vi "Dequeue Published Result by Type.vi"(8 "error in (no error)":errorcluster, 9 "timeout in ms":i32, 10 "Result Type":T1, 11 "Mock Result Observer In":refnum<class "Mock Result Observer.lvclass">) -> (0 "error out":errorcluster, 1 "timed out?":bool, 2 "Result":T2={"Name"="", "Message"="", "Description"="", "Status"=enum."Passed", "Result Type"=enum."Method", "Execution Time"=0.0}, 3 "Mock Result Observer Out":refnum<class "Mock Result Observer.lvclass">)   [LabVIEW 2020, in "Mock Result Observer.lvclass"]
uses:
  Mock Result Observer.lvclass
  Core/Result/Result.ctl
  Core/Result/Status.ctl
  Core/Result/Type.ctl
  Core/Result/Result.lvlib
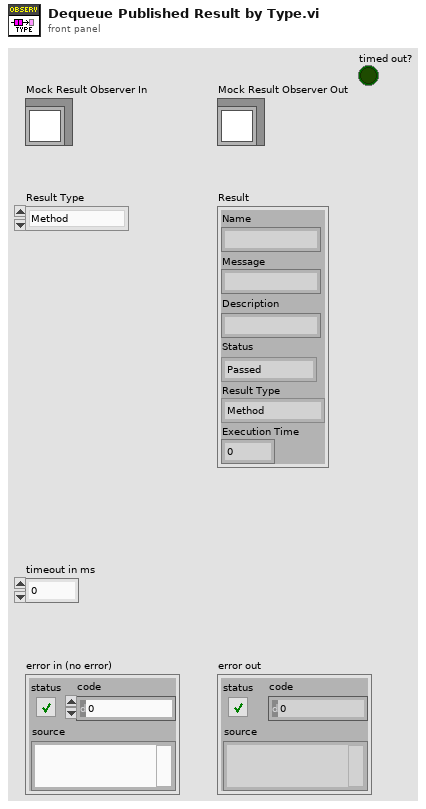
[diagram p1: front panel]
types:
  T1 = typedef "Result.lvlib/Type.ctl" = enum16{"Method", "Case", "Suite", "Pass", "Fail", "Skip", "Pass if", "Fail if", "Pass if Error", "Fail if Error", "Pass if Equal", "Fail if Equal"}
  T2 = typedef "Result.lvlib/Result.ctl" = cluster{"Name":string, "Message":string, "Description":string, "Status":T3, "Result Type":T1, "Execution Time":dbl}
  T3 = typedef "Result.lvlib/Status.ctl" = enum16{"", "Passed", "Failed", "Error", "Skipped", "Setup Error", "Broken", "Teardown Error"}
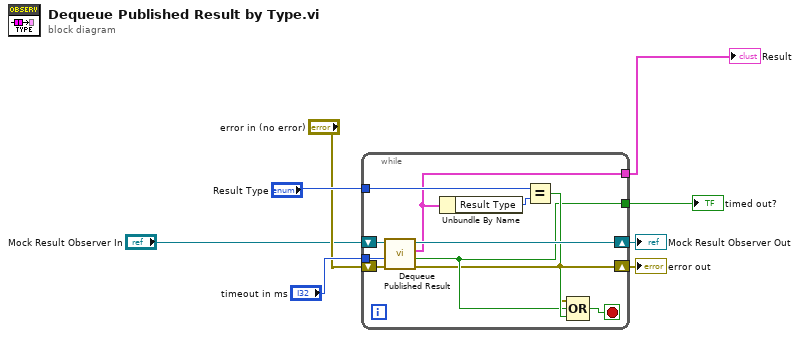
[diagram p0: block diagram]
diagram:
  n1 = while {
    tunnel: "timeout in ms" -> [w16]
    shift-right: [w19] -> w2
    shift-left: "Mock Result Observer In" -> [w18]
    shift-right: [w9] -> w3
    shift-left: "error in (no error)" -> [w17]
    tunnel: "Result Type" -> [w15]
    tunnel: [w11] -> w8
    tunnel: [w10] -> w1
    stop <- w13 stop-if-true
    n2 = call "Dequeue Published Result.vi"("error in (no error)"=w17, "timeout in ms (-1)"=w16, "Mock Result Observer In"=w18) -> ("error out"=w9:errorcluster, "timed out?"=w10:bool, "Result"=w11:T2, "Mock Result Observer Out"=w19:refnum<class "Mock Result Observer.lvclass">)  [unwired: 5 in]
    n3 = Unbundle By Name(w11) -> ("Result Type"=w14:T1)
    n4 = Equal?(x=w15, y=w14) -> (x = y?=w12:bool)
    n5 = Compound Arithmetic op=OR(w9, w10, w12) -> (w13:bool)
  }
  "Result" <- w8
  "error out" <- w3
  "Mock Result Observer Out" <- w2
  "timed out?" <- w1
